vi "IniPara.vi"(8 "error in":errorcluster, 10 "Para section":string="Para", 11 "INI file path":path=path "D:/ZDX201 塗膠螺絲鎖固自動化_鴻海/ZDX201_LabView/iniData/Para_iniData.ini") -> (0 "PLC mode":bool=TRUE, 1 "開發模式":bool=TRUE, 2 "Pass下料區":bool=TRUE, 3 "value":bool, 4 "error out":errorcluster, 5 "MoveCurve":bool, 6 "一律放行":bool)   [LabVIEW 2019]
uses:
  <vilib>/Utility/config.llb/Read Key (Boolean).vi
  <vilib>/Utility/config.llb/NI_LVConfig.lvlib
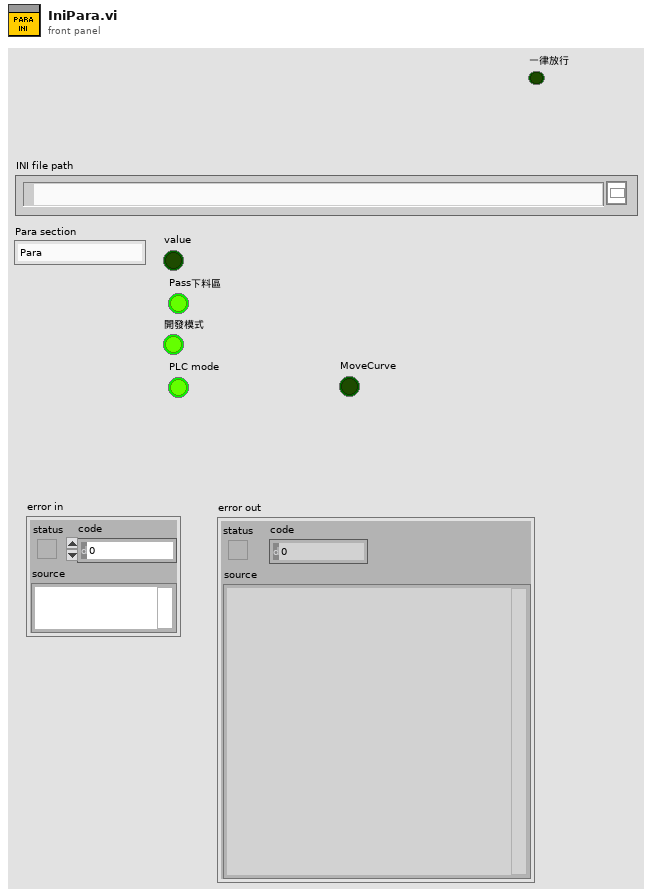
[diagram p1: front panel]
types:
  T1 = typedef "NI_LVConfig.lvlib/Config Data RefNum.ctl" = refnum<k1>
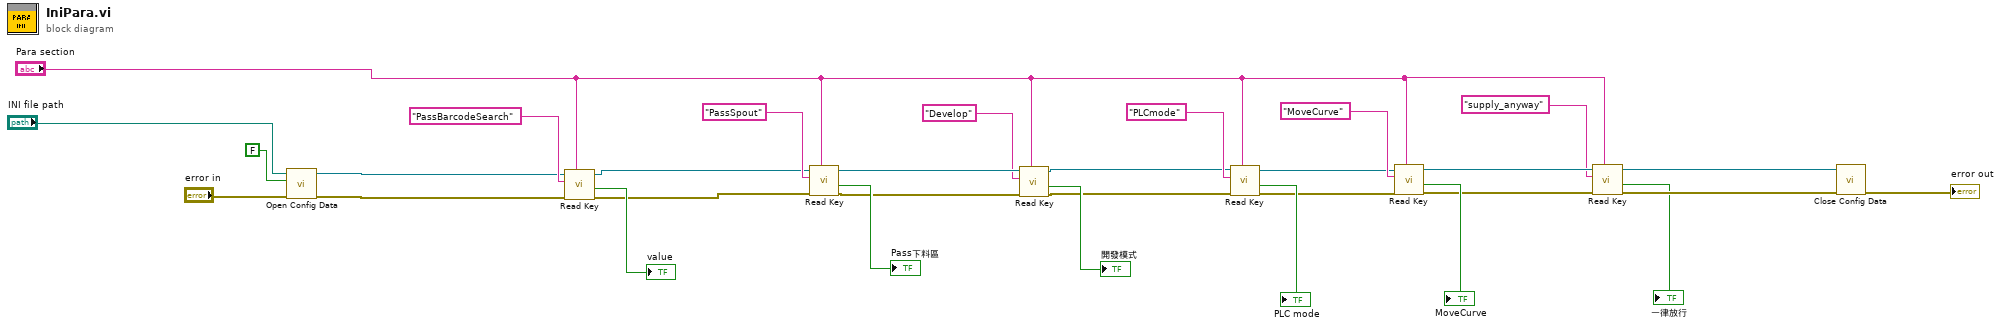
[diagram p0: block diagram]
diagram:
  n1 = call <vilib>:"Open Config Data.vi"("error in (no error)"="error in", "create file if necessary (T)"=FALSE ("create file if necessary? (T)"), "configuration file path"="INI file path") -> ("error out"=w24:errorcluster, "refnum"=w25:T1)  [unwired: 6 in, 1 out]
  n2 = call-poly <vilib>:"Read Key.vi"("section"="Para section", "error in (no error)"=w24, "key"="PassBarcodeSearch", "refnum"=w25) -> ("error out"=w20:errorcluster, "value"=→"value":bool, "refnum out"=w21:T1)  [unwired: 1 in, 4 out]
  n3 = call-poly <vilib>:"Read Key.vi"("section"="Para section", "error in (no error)"=w20, "key"="PassSpout", "refnum"=w21) -> ("error out"=w17:errorcluster, "value"=→"Pass下料區":bool, "refnum out"=w18:T1)  [unwired: 1 in, 4 out]
  n4 = call-poly <vilib>:"Read Key.vi"("section"="Para section", "error in (no error)"=w17, "key"="Develop", "refnum"=w18) -> ("error out"=w13:errorcluster, "value"=→"開發模式":bool, "refnum out"=w14:T1)  [unwired: 1 in, 4 out]
  n5 = call-poly <vilib>:"Read Key.vi"("section"="Para section", "error in (no error)"=w13, "key"="PLCmode", "refnum"=w14) -> ("error out"=w8:errorcluster, "value"=→"PLC mode":bool, "refnum out"=w9:T1)  [unwired: 1 in, 4 out]
  n6 = call-poly <vilib>:"Read Key.vi"("section"="Para section", "error in (no error)"=w8, "key"="MoveCurve", "refnum"=w9) -> ("error out"=w5:errorcluster, "value"=→"MoveCurve":bool, "refnum out"=w6:T1)  [unwired: 1 in, 4 out]
  n7 = call-poly <vilib>:"Read Key.vi"("section"="Para section", "error in (no error)"=w5, "key"="supply_anyway", "refnum"=w6) -> ("error out"=w3:errorcluster, "value"=→"一律放行":bool, "refnum out"=w4:T1)  [unwired: 1 in, 4 out]
  n8 = call <vilib>:"Close Config Data.vi"("error in (no error)"=w3, "refnum"=w4) -> ("error out"=→"error out":errorcluster)  [unwired: 1 in, 8 out]
